vi "CleanUp.vi"(0 "object in":refnum<class "Client.lvclass">, 5 "Error In":errorcluster) -> (14 "object out":refnum<class "Client.lvclass">, 19 "Error Out":errorcluster)   [LabVIEW 2024, in "Client.lvclass"]
uses:
  Client.lvclass
  Client.lvclass/Client.ctl
  Abstractions/DataType/DataType.lvclass
panel:
  # "Connector Pane"
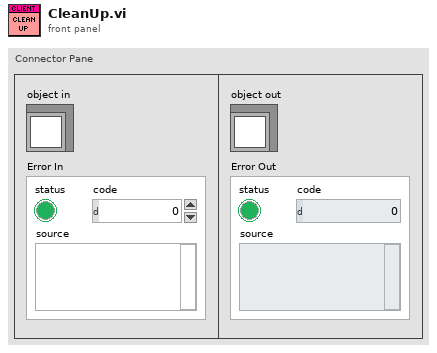
[diagram p1: front panel]
types:
  T1 = typedef "File Type.ctl" = enum32{"TDMS", "EXCEL"}
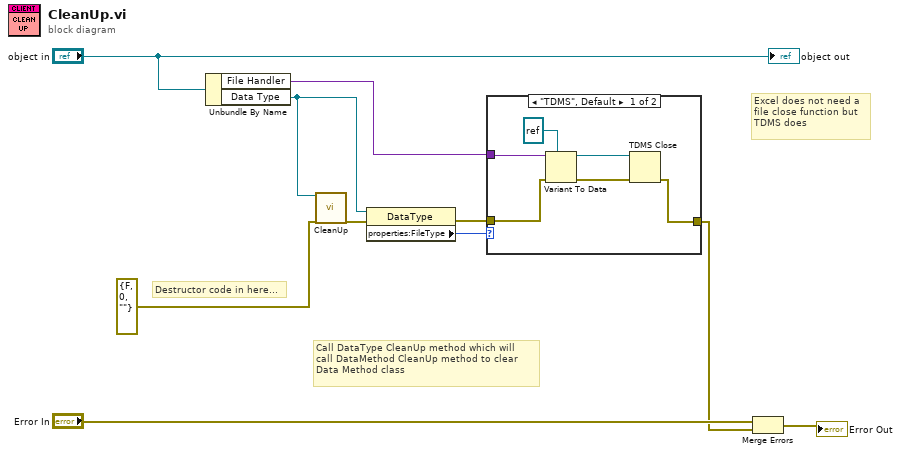
[diagram p0: block diagram]
diagram:
  # "Call DataType CleanUp method which will\ncall DataMethod CleanUp method to clear\nData Method class"
  # "Excel does not need a\nfile close function but\nTDMS does"
  # "Destructor code in here..."
  n1 = Unbundle By Name("object in") -> ("File Handler"=w4:variant, "Data Type"=w6:refnum<class "DataType.lvclass">)
  n2 = call-dynamic "CleanUp.vi"("object in"=w6, "error in (no error)"=errorcluster {"status"=FALSE, "code"=0, "source"=""}) -> ("error out"=w3:errorcluster)  [unwired: 16 in, 1 out]
  n3 = property class="DataType"(reference=w6, error in=w3) -> (error out=w2:errorcluster, "properties:FileType"=w5:T1)  [unwired: 1 out]
  n4 = case shown="\"TDMS\", Default" w5 {
    tunnel: w4 -> [w16 _]
    tunnel: w2 -> [w12 w17]
    tunnel: [w11 w17] -> w1
    frame "TDMS", Default {
      n5 = Variant To Data(error in=w12, type=refnum<k34> refnum ("tdms file"), Variant=w16) -> (data=w14:refnum<k34>, error out=w13:errorcluster)
      n6 = TDMS Close(8:w13, 11:w14) -> (0:w11:errorcluster)  [unwired: 1 out]
    }
    frame "EXCEL" {
    }
  }
  n7 = Merge Errors("Error In", w1) -> (→"Error Out":errorcluster)
  "object out" <- "object in"
